vi "niRFSTS Sequence Flow Create Sequence File.vi"(0 "Session Handle in":T1, 5 "Sequence File Path":path, 9 "Template Path":path, 11 "error in (no error)":errorcluster, 12 "From Template?":bool) -> (4 "Session Handle out":T1, 15 "error out":errorcluster)   [LabVIEW 2018, in "niRFSTS Sequence Flow.lvclass"]
uses:
  niRFSTS Sequence Flow.lvclass
  Typedefs/Session Handle.ctl
  niRFSTS Sequence Flow.lvclass/niRFSTS Sequence Flow.ctl
  Plugins/TestStand API Tools (TSAT).lvlibp/Sequence File Actions/TSAT Sequence File Actions.lvlib
  Plugins/TestStand API Tools (TSAT).lvlibp/TSAT Examples/TSAT Examples.lvlib
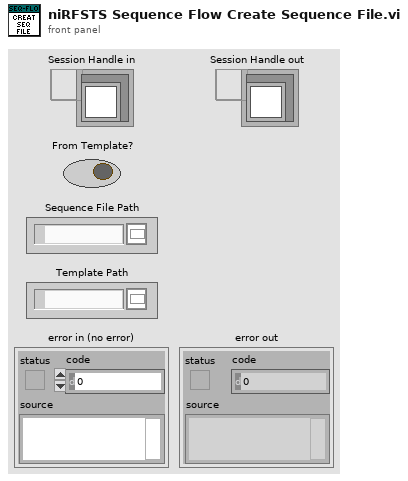
[diagram p1: front panel]
types:
  T1 = typedef "niRFSTS Sequence Flow.lvclass/Session Handle.ctl" = refnum<data-value>
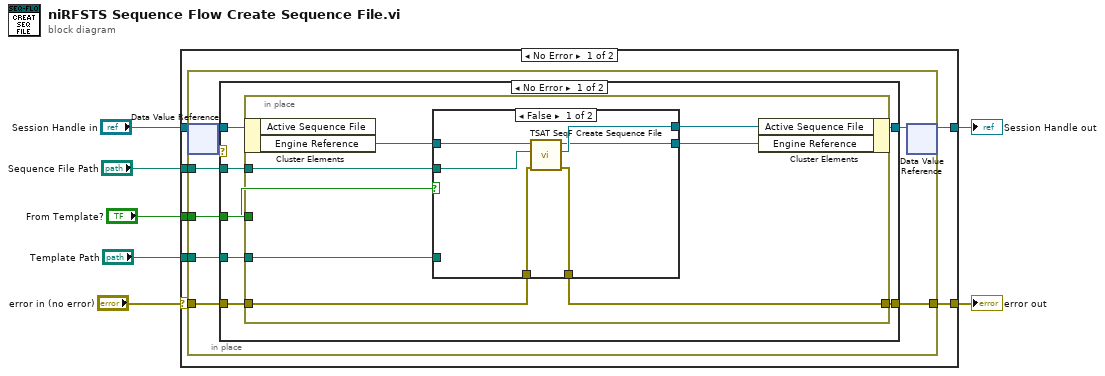
[diagram p0: block diagram]
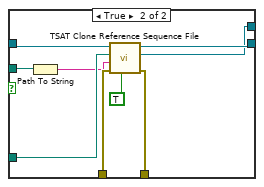
[diagram p2: hidden frame]
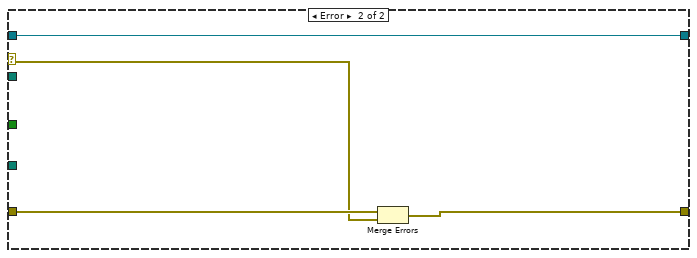
[diagram p3: hidden frame]
diagram:
  n1 = case shown="No Error" "error in (no error)" {
    selector: "error in (no error)" -> [w12 w57]
    tunnel: "Session Handle in" -> [w14 w58]
    tunnel: [w13 w58] -> w6
    tunnel: [w11 w57] -> w5
    tunnel: "Sequence File Path" -> [w10 _]
    tunnel: "From Template?" -> [w9 _]
    tunnel: "Template Path" -> [w8 _]
    frame No Error {
      n2 = in-place {
        in-place-border: w12 -> [w18]
        in-place-border: [w21] -> w11
        in-place-border: w10 -> [w17]
        in-place-border: w9 -> [w16]
        in-place-border: w8 -> [w15]
        n3 = in-place-dvr #1(w14) -> (w22:refnum<class "niRFSTS Sequence Flow.lvclass">, w19:errorcluster)
        n4 = case shown="No Error" w19 {
          selector: w19 -> [_ w55]
          tunnel: w22 -> [w29 w53]
          tunnel: [w28 w54] -> w21
          tunnel: [w27 w53] -> w20
          tunnel: w18 -> [w26 w56]
          tunnel: w17 -> [w25 _]
          tunnel: w16 -> [w24 _]
          tunnel: w15 -> [w23 _]
          frame No Error {
            n5 = in-place {
              in-place-border: [w34] -> w28
              in-place-border: w26 -> [w35]
              in-place-border: w25 -> [w36]
              in-place-border: w24 -> [w31]
              in-place-border: w23 -> [w30]
              n6 = in-place-cluster #2(w29) -> ("Engine Reference"=w37:refnum<k7>)  [unwired: 1 out]
              n7 = case shown="False" w31 {
                tunnel: w37 -> [w43 w52]
                tunnel: w36 -> [w42 w45]
                tunnel: w35 -> [w41 w50]
                tunnel: [w40 w49] -> w34
                tunnel: [w39 w47] -> w33
                tunnel: [w38 w48] -> w32
                tunnel: w30 -> [_ w51]
                frame False {
                  n8 = call "TSAT SeqF Create Sequence File.vi"("Error In"=w41, "Sequence File Location"=w42, "Engine In"=w43) -> ("Error Out"=w40:errorcluster, "Sequence File"=w39:refnum<k7>, "Engine Out"=w38:refnum<k7>)  [unwired: 6 in]
                }
                frame True {
                  n9 = Path To String(path=w45) -> (string=w44:string)
                  n10 = call "TSAT Clone Reference Sequence File.vi"("Specify Path"=TRUE, "Error In"=w50, "New File Name"=w44, "Sequence File Path"=w51, "Engine In"=w52) -> ("Error Out"=w49:errorcluster, "New Sequence File Out"=w47:refnum<k7>, "Engine out"=w48:refnum<k7>)  [unwired: 4 in]
                }
              }
              n11 = in-place-cluster #2("Active Sequence File"=w33, "Engine Reference"=w32) -> (w27:refnum<class "niRFSTS Sequence Flow.lvclass">)
            }
          }
          frame Error {
            n12 = Merge Errors(w56, w55) -> (w54:errorcluster)
          }
        }
        n13 = in-place-dvr #1(w20) -> (w13:T1)  [unwired: 1 out]
      }
    }
    frame Error {
    }
  }
  "Session Handle out" <- w6
  "error out" <- w5
